vi "Flicker Data Acquisition - Main.vi"() -> ()   [LabVIEW 2013]
panel:
  in  "Sphere":u16(ring) items=["1m", "2m (naked)", "2m (jacketed)"]
  in  "Notes (plain text, no commas)":string
  in  "Amp gain":string
  in  "Test repeat #":string
  in  "Dim level% (3 sig fig)\n(\"100\" if no dimming)":string
  in  "Dimmer description\n(\"power supply\" for no\ndimming)":string
  in  "Model (eg. \"omni05\")":string
  out "appended path":path
  out "data":waveform(dbl)(graph)
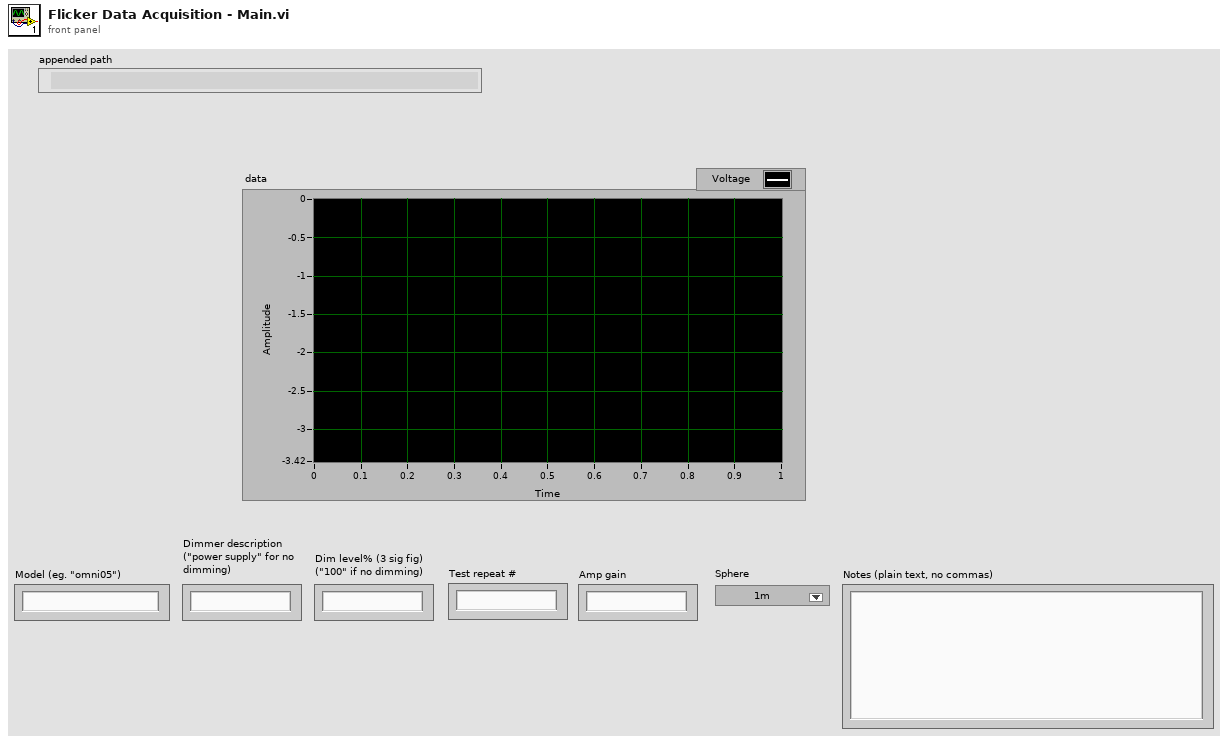
[diagram p1: front panel]
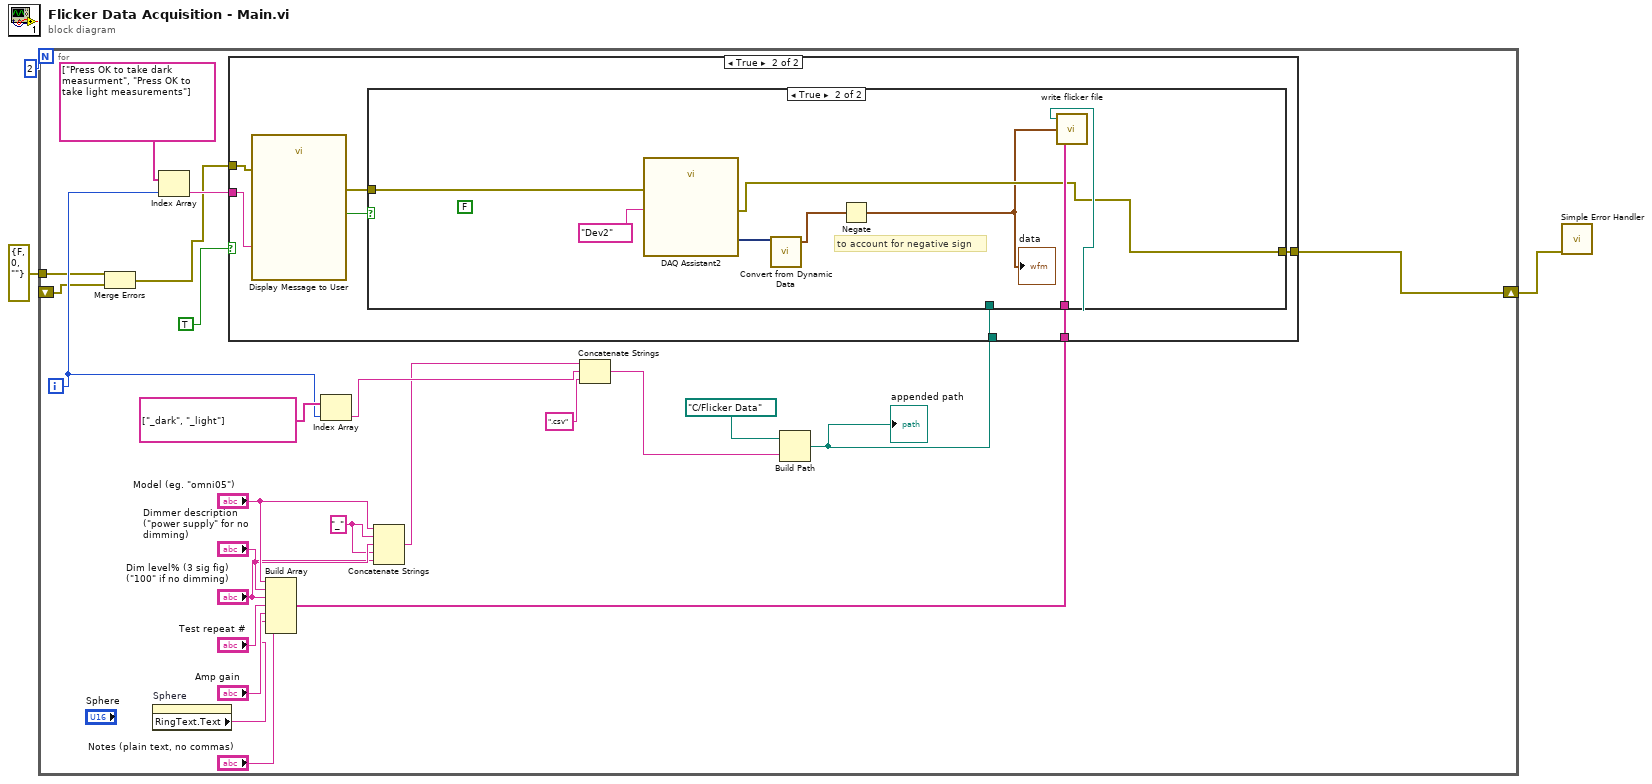
[diagram p0: block diagram]
diagram:
  n1 = for {
    N: 2 -> [_]
    tunnel: errorcluster {"status"=FALSE, "code"=0, "source"=""} ("error out") -> [w7]
    shift-right: [w9] -> w2
    shift-left: _ -> [w6]
    i -> [w22]
    w14 = "_"
    n2 = Merge Errors(w7, w6) -> (w8:errorcluster)
    n3 = property on="Sphere" class="Ring (strict)"() -> ("RingText.Text"=w4:string)  [unwired: 2 in, 2 out]
    n4 = Index Array(array=string[] ["Press OK to take dark measurment", "Press OK to take light measurements"], index=w22) -> (element=w26:string)
    n5 = Build Array("Model (eg. \"omni05\")", "Dimmer description\n(\"power supply\" for no\ndimming)", "Dim level% (3 sig fig)\n(\"100\" if no dimming)", "Test repeat #", "Amp gain", w4, "Notes (plain text, no commas)") -> (w11:string[])
    n6 = Index Array(array=string[] ["_dark", "_light"], index=w22) -> (element=w20:string)
    n7 = Concatenate Strings("Model (eg. \"omni05\")", w14, "Dimmer description\n(\"power supply\" for no\ndimming)", w14, "Dim level% (3 sig fig)\n(\"100\" if no dimming)") -> (w12:string)
    n8 = Concatenate Strings(w12, w20, ".csv" ("string")) -> (w25:string)
    n9 = Build Path(base path=path "C:/Flicker Data", name or relative path=w25) -> (appended path=w24:path)
    "appended path" <- w24
    n10 = case shown="True" TRUE {
      tunnel: w26 -> [_ w33]
      tunnel: w24 -> [_ w32]
      tunnel: w8 -> [w28 w31]
      tunnel: w11 -> [_ w30]
      tunnel: [w28 w29] -> w9
      frame False {
      }
      frame True {
        n11 = call "Display Message to User"("error in (no error)"=w31, "Message"=w33) -> ("error out"=w35:errorcluster, "OK"=w34:bool)  [unwired: 8 in]
        n12 = case shown="True" w34 {
          tunnel: w35 -> [w36 w41]
          tunnel: w32 -> [_ w43]
          tunnel: w30 -> [_ w44]
          tunnel: [w36 w40] -> w29
          frame False {
          }
          frame True {
            (unwired) FALSE
            # "to account for negative sign"
            n13 = call "DAQ Assistant2"("error in"=w41, "device name"=tag "Dev2") -> ("data"=w42:dynamicdata, "error out"=w40:errorcluster)  [unwired: 15 in, 1 out]
            n14 = call "Convert from Dynamic Data"("Dynamic Data Type"=w42) -> ("Waveform"=w38:waveform(dbl))  [unwired: 3 in]
            n15 = Negate(x=w38) -> (-x=w37:waveform(dbl))
            "data" <- w37
            n16 = call "write flicker file.vi"("Array"=w44, "Waveform Data"=w37, "appended path"=w43) -> ()  [unwired: 1 in]
          }
        }
      }
    }
  }
  n17 = call <vilib>:"Simple Error Handler.vi"("error in (no error)"=w2) -> ()  [unwired: 4 in, 5 out]
